vi "Intialize_GamryRef600.vi"() -> ()   [LabVIEW 2023]
panel:
  out "Potentiostat Model":string
  out "error out":errorcluster
  in  "GAMRYCOMLib.IGamryPstat":refnum<k7>
  in  "GAMRYCOMLib.IGamryDeviceList":refnum<k7>
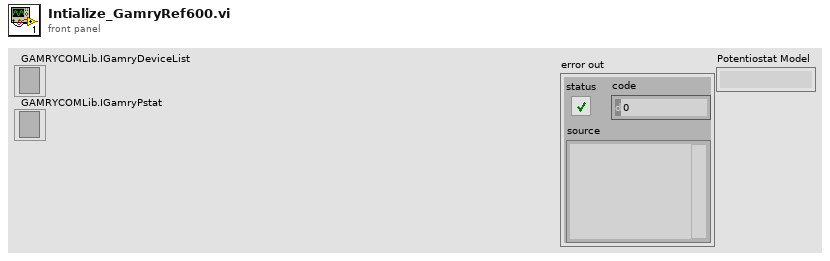
[diagram p1: front panel]
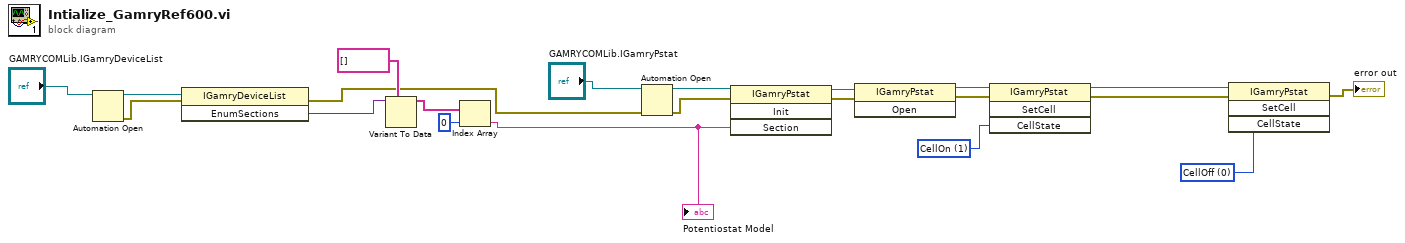
[diagram p0: block diagram]
diagram:
  w3 = 0 items=["CellOff", "CellOn", "CellMon", "CellRelay"] ("CellState")
  w5 = 1 items=["CellOff", "CellOn", "CellMon", "CellRelay"] ("CellState")
  n1 = Automation Open(Automation Refnum="GAMRYCOMLib.IGamryDeviceList") -> (Automation Refnum=w20:refnum<k7>, error out=w19:errorcluster)  [unwired: 3 in]
  n2 = invoke class="IGamryDeviceList" method="EnumSections"(reference=w20, error in=w19) -> (error out=w13:errorcluster, "EnumSections"=w18:variant)  [unwired: 1 in, 1 out]
  n3 = Variant To Data(type=string[] [], Variant=w18) -> (data=w16:string[])  [unwired: 1 in, 1 out]
  n4 = Index Array(array=w16, index=0) -> (element=w11:string)
  "Potentiostat Model" <- w11
  n5 = Automation Open(error in (no error)=w13, Automation Refnum="GAMRYCOMLib.IGamryPstat") -> (Automation Refnum=w12:refnum<k7>, error out=w9:errorcluster)  [unwired: 2 in]
  n6 = invoke class="IGamryPstat" method="Init"(reference=w12, error in=w9, "Section"=w11) -> (reference out=w10:refnum<k7>, error out=w8:errorcluster)  [unwired: 1 in, 2 out]
  n7 = invoke class="IGamryPstat" method="Open"(reference=w10, error in=w8) -> (reference out=w7:refnum<k7>, error out=w6:errorcluster)  [unwired: 1 in, 1 out]
  n8 = invoke class="IGamryPstat" method="SetCell"(reference=w7, error in=w6, "CellState"=w5) -> (reference out=w2:refnum<k7>, error out=w1:errorcluster)  [unwired: 1 in, 2 out]
  n9 = invoke class="IGamryPstat" method="SetCell"(reference=w2, error in=w1, "CellState"=w3) -> (error out=→"error out":errorcluster)  [unwired: 1 in, 3 out]
